vi "Conv_Deg_Radians.vi"(10 "Degress":dbl) -> (2 "Radians":dbl)   [LabVIEW 2019, in "PathExecution_Library.lvlib"]
doc: "Convert Feet to Meters"
uses:
  PathExecution_Library.lvlib
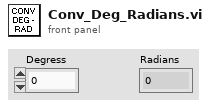
[diagram p1: front panel]
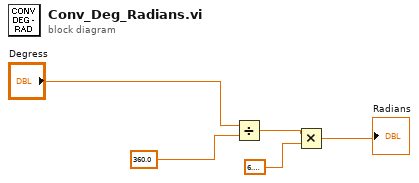
[diagram p0: block diagram]
diagram:
  n1 = Divide(x="Degress", y=360.0) -> (x/y=w3:dbl)
  n2 = Multiply(x=w3, y=6.283185307179586) -> (x*y=→"Radians":dbl)
